vi "Message Notifier.vi"(8 "error in":errorcluster, 10 "Notifier Data":T1, 11 "Main Data Buffer In":T3) -> (0 "error out":errorcluster, 3 "Main Data Buffer Out":T3)   [LabVIEW 2020, in "SECS Bridge.lvlib"]
uses:
  SECS Bridge.lvlib
  Main Data Buffer.ctl
  SECS Communication/HSMS Class/HSMS Class.lvclass
  SECS Communication/SECS Data Class/SECS Data Class.lvclass
  SECS Scenarios/Scenarios Class/Scenarios Class.lvclass
  SECS Communication/HSMS Class/Notifier Data.ctl
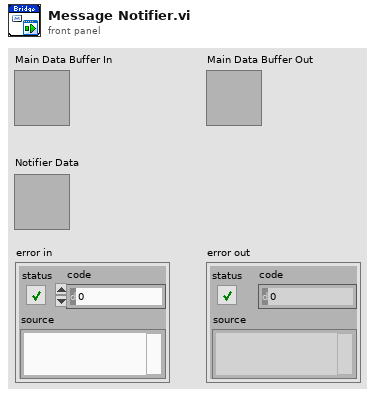
[diagram p1: front panel]
types:
  T1 = typedef "SECS Communication.lvlib/HSMS Class.lvclass/Notifier Data.ctl" = cluster{"Notifier Type":T2, "Data":variant, "Time":timestamp}
  T2 = typedef "SECS Communication.lvlib/HSMS Class.lvclass/Notifier Type.ctl" = enum16{"TCPIP Connect", "TCPIP Disconnect", "Receive Message", "Send Message", "T3 Timeout", "T6 Timeout", "T7 Timeout", "Error", "Stop"}
  T3 = typedef "SECS Bridge.lvlib/Main Data Buffer.ctl" = cluster{"HSMS Class":refnum<class "HSMS Class.lvclass">, "SECS Data Class":refnum<class "SECS Data Class.lvclass">, "Scenarios Class":refnum<class "Scenarios Class.lvclass">, "VI Refnum":refnum<vi>, "Ctl Refnum Map":map{string, refnum<vi>}, "Timeout":i32, "Notifier Data":string[], "Event Refnum":refnum<event-registration>}
  T4 = typedef "SECS Bridge.lvlib/Broadcast Refnum.ctl" = cluster{"Nottifier Data User Event":refnum<user-event>, "HSMS State User Event":refnum<user-event>, "On-Line User Event":refnum<user-event>}
  T5 = enum32{"Invalid", "Standard", "Closed", "Hidden", "Minimized", "Maximized"}
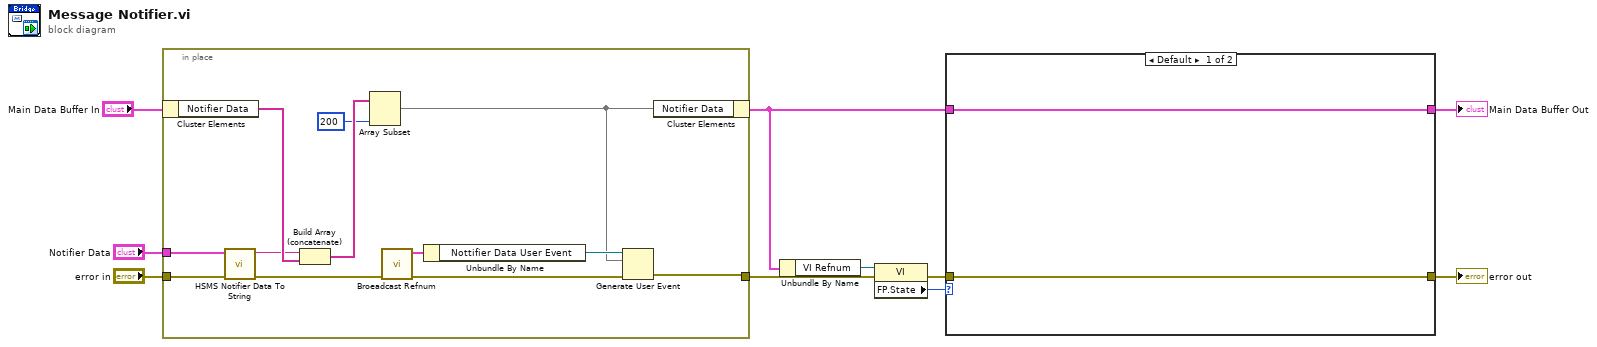
[diagram p0: block diagram]
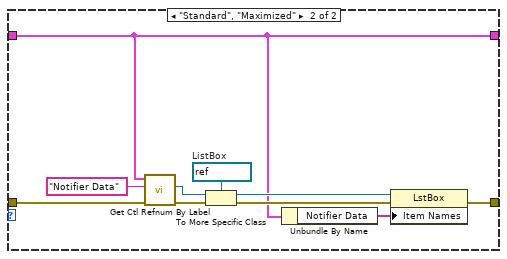
[diagram p2: hidden frame]
diagram:
  n1 = in-place {
    in-place-border: "error in" -> [w22]
    in-place-border: "Notifier Data" -> [w21]
    in-place-border: [w12] -> w5
    n2 = in-place-cluster #1("Main Data Buffer In") -> ("Notifier Data"=w20:string[])
    n3 = call "HSMS Notifier Data To String.vi"("error in (no error)"=w22, "Notifier Data"=w21) -> ("error out"=w16:errorcluster, "String"=w19:string)  [unwired: 8 in]
    n4 = Build Array (concatenate)(w19, w20) -> (w18:string[])
    n5 = Array Subset(array=w18, length=200) -> (w11:string[])  [unwired: 1 in]
    n6 = call "Broeadcast Refnum.vi"("error in"=w16) -> ("error out"=w14:errorcluster, "Broadcast Refnum"=w15:T4)  [unwired: 9 in]
    n7 = Unbundle By Name(w15) -> ("Nottifier Data User Event"=w13:refnum<user-event>)
    n8 = Generate User Event(user event=w13, event data cluster=w11, error in=w14) -> (error out=w12:errorcluster)  [unwired: 1 in, 1 out]
    n9 = in-place-cluster #1("Notifier Data"=w11) -> (w6:T3)
  }
  n10 = Unbundle By Name(w6) -> ("VI Refnum"=w4:refnum<vi>)
  n11 = property class="VI"(reference=w4, error in=w5) -> (error out=w3:errorcluster, "FP.State"=w2:T5)  [unwired: 1 out]
  n12 = case shown="Default" w2 {
    tunnel: [w23 w28] -> w7
    tunnel: w6 -> [w24 w25]
    tunnel: w3 -> [w23 w26]
    tunnel: [w24 w25] -> w1
    frame Default {
    }
    frame "Standard", "Maximized" {
      w31 = refnum<vi> refnum  # ListBox
      n13 = call "Get Ctl Refnum By Label.vi"("error in"=w26, "Label"="Notifier Data", "Main Data Buffer In"=w25) -> ("error out"=w33:errorcluster, "Ctl Refnum"=w32:refnum<vi>)  [unwired: 6 in, 1 out]
      n14 = To More Specific Class(target class=w31, reference=w32, error in=w33) -> (specific class reference=w29:refnum<vi>, error out=w30:errorcluster)
      n15 = Unbundle By Name(w25) -> ("Notifier Data"=w27:string[])
      n16 = property class="LstBox"(reference=w29, error in=w30, "Item Names"=w27) -> (error out=w28:errorcluster)  [unwired: 1 out]
    }
  }
  "error out" <- w7
  "Main Data Buffer Out" <- w1
